vi "WriteToINIFile.vi"(8 "error in (no error)":errorcluster, 10 "Refnum in":T1, 11 "SiemensDigitalEnergyMeter in":refnum<class "SiemensDigitalEnergyMeter.lvclass">) -> (0 "error out":errorcluster, 3 "SiemensDigitalEnergyMeter out":refnum<class "SiemensDigitalEnergyMeter.lvclass">)   [LabVIEW 2018, in "SensorPlugins.lvlib" / "SiemensDigitalEnergyMeter.lvclass"]
doc: "This VI writes the configuration to the INI file."
uses:
  SiemensDigitalEnergyMeter.lvclass
  <vilib>/Utility/config.llb/Config Data RefNum.ctl
  <vilib>/Utility/config.llb/NI_LVConfig.lvlib
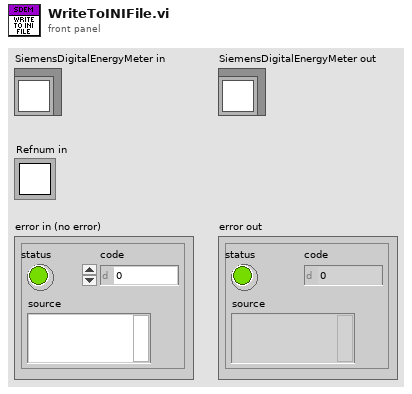
[diagram p1: front panel]
types:
  T1 = typedef "NI_LVConfig.lvlib/Config Data RefNum.ctl" = refnum<k1>
  T2 = typedef "SensorPlugins.lvlib/SiemensDigitalEnergyMeter.lvclass/SiemensDigitalEnergyMeterControls.ctl" = cluster{"Measurement(s)":u16[], "IP Address":string, "Port (502)":u16, "Configuration Commands":string, "Use Measurement Commands Text Box?":bool, "Measurement Commands":string, "Connected?":bool, "Serial Number":string}[]
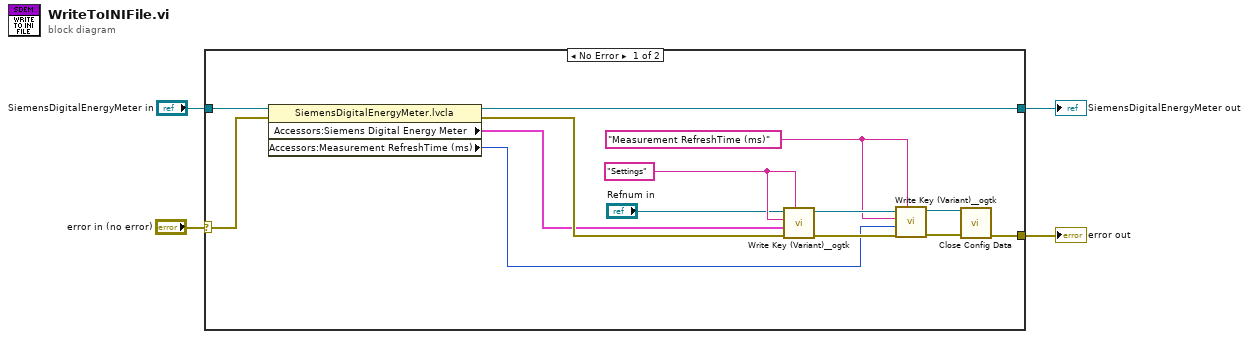
[diagram p0: block diagram]
diagram:
  n1 = case shown="No Error" "error in (no error)" {
    selector: "error in (no error)" -> [w16 w20]
    tunnel: "SiemensDigitalEnergyMeter in" -> [w17 w19]
    tunnel: [w15 w19] -> w2
    tunnel: [w11 w20] -> w1
    frame No Error {
      w6 = "Measurement RefreshTime (ms)" ("section (optional)")
      w18 = "Settings" ("section (optional)")
      n2 = property class="SiemensDigitalEnergyMeter.lvcla"(reference=w17, error in=w16) -> (reference out=w15:refnum<class "SiemensDigitalEnergyMeter.lvclass">, error out=w14:errorcluster, "Accessors:Siemens Digital Energy Meter"=w13:T2, "Accessors:Measurement RefreshTime (ms)"=w5:u32)
      n3 = call <userlib>:"Write Key (Variant)__ogtk.vi"("section"=w18, "error in (no error)"=w14, "key-value"=w13, "key (optional)"=w18, "refnum"="Refnum in") -> ("error out"=w10:errorcluster, "refnum out"=w7:T1)  [unwired: 5 in]
      n4 = call <userlib>:"Write Key (Variant)__ogtk.vi"("section"=w6, "error in (no error)"=w10, "key-value"=w5, "key (optional)"=w6, "refnum"=w7) -> ("error out"=w9:errorcluster, "refnum out"=w8:T1)  [unwired: 5 in]
      n5 = call <vilib>:"Close Config Data.vi"("error in (no error)"=w9, "refnum"=w8) -> ("error out"=w11:errorcluster)  [unwired: 8 in, 1 out]
    }
    frame Error {
    }
  }
  "error out" <- w1
  "SiemensDigitalEnergyMeter out" <- w2
